vi "AB_Engine_Update_INI_Header.vi"(8 "error in (no error)":errorcluster, 9 "Old INI Name":string, 10 "Application Name w/o extension":string, 11 "Path to INI":path) -> (0 "error out":errorcluster, 3 "Path to INI out":path)   [LabVIEW 2020]
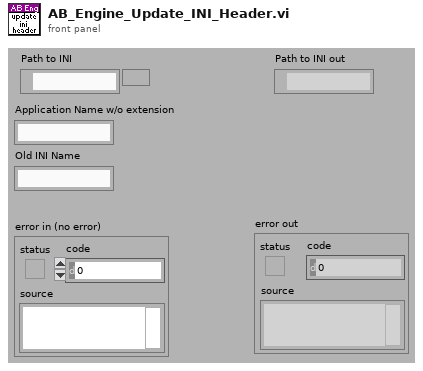
[diagram p1: front panel]
types:
  T1 = enum16{"open", "replace", "create", "open or create", "replace or create", "replace or create with confirmation"}
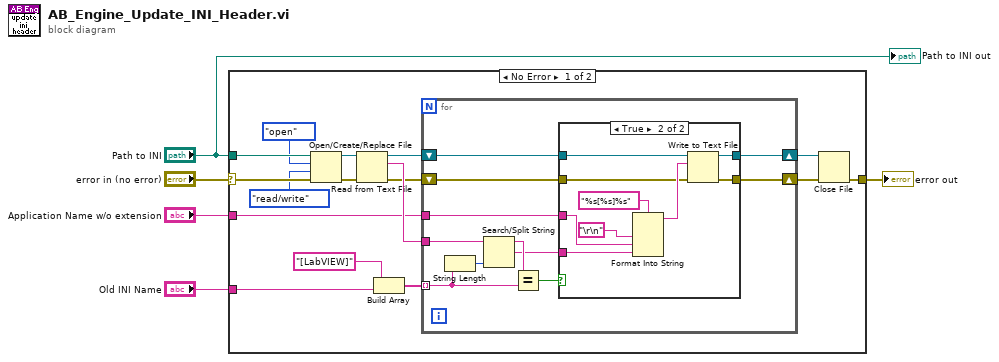
[diagram p0: block diagram]
diagram:
  n1 = case shown="No Error" "error in (no error)" {
    selector: "error in (no error)" -> [w8 w44]
    tunnel: "Old INI Name" -> [w18 _]
    tunnel: "Application Name w/o extension" -> [w15 _]
    tunnel: "Path to INI" -> [w11 _]
    tunnel: [w12 w44] -> w3
    frame No Error {
      n2 = Open/Create/Replace File(file path (use dialog)=w11, error in=w8, operation (0:open)=T1."open", access (0:read/write)=enum16{"read/write", "read-only", "write-only"}."read/write") -> (refnum out=w10:refnum<file>, error out=w9:errorcluster)  [unwired: 2 in, 1 out]
      n3 = Read from Text File(file (use dialog)=w10, error in=w9) -> (refnum out=w20:refnum<file>, text=w21:string, error out=w14:errorcluster)  [unwired: 2 in, 1 out]
      n4 = Build Array("[LabVIEW]", w18) -> (w16:string[])
      n5 = for {
        tunnel: w21 -> [w30]
        tunnel: w16 -> [w29] mode=indexing
        shift-right: [w26] -> w19
        shift-left: w20 -> [w28]
        tunnel: w15 -> [w24]
        shift-right: [w22] -> w13
        shift-left: w14 -> [w23]
        n6 = String Length(string=w29) -> (length=w31:i32)
        n7 = Search/Split String(string=w30, offset (0)=w31) -> (substring before match=w32:string, match + rest of string=w27:string)  [unwired: 1 in, 1 out]
        n8 = Equal?(x=w32, y=w29) -> (x = y?=w25:bool)
        n9 = case shown="True" w25 {
          tunnel: w28 -> [w34 w42]
          tunnel: w27 -> [_ w37]
          tunnel: [w34 w41] -> w26
          tunnel: w24 -> [_ w36]
          tunnel: w23 -> [w33 w39]
          tunnel: [w33 w38] -> w22
          frame False {
          }
          frame True {
            n10 = Format Into String(format string="%s[%s]%s", "\r\n", w36, w37) -> (resulting string=w40:string)  [unwired: 2 in, 1 out]
            n11 = Write to Text File(file (use dialog)=w42, text=w40, error in=w39) -> (refnum out=w41:refnum<file>, error out=w38:errorcluster)  [unwired: 1 in, 1 out]
          }
        }
      }
      n12 = Close File(refnum=w19, error in=w13) -> (error out=w12:errorcluster)  [unwired: 1 out]
    }
    frame Error {
    }
  }
  "error out" <- w3
  "Path to INI out" <- "Path to INI"
